vi "SaveForPrevious.vi"() -> ()   [LabVIEW 2016]
panel:
  out "error out":errorcluster
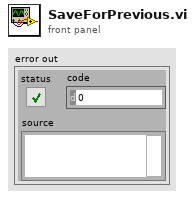
[diagram p1: front panel]
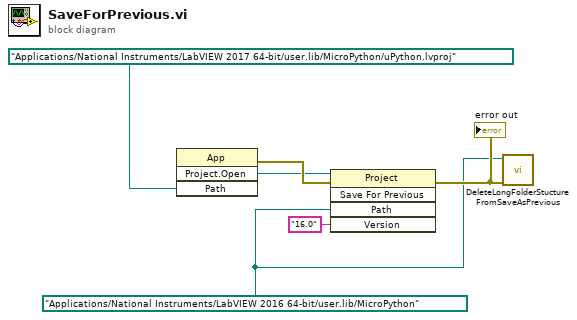
[diagram p0: block diagram]
diagram:
  w4 = path "/Applications/National Instruments/LabVIEW 2016 64-bit/user.lib/MicroPython" ("Path")
  n1 = invoke class="App" method="Project.Open"("Path"=path "/Applications/National Instruments/LabVIEW 2017 64-bit/user.lib/MicroPython/uPython.lvproj") -> (error out=w3:errorcluster, "Project:Open"=w2:refnum<vi>)  [unwired: 3 in, 2 out]
  n2 = invoke class="Project" method="Save For Previous"(reference=w2, error in=w3, "Path"=w4, "Version"="16.0") -> (error out=w5:errorcluster)  [unwired: 1 in, 4 out]
  "error out" <- w5
  n3 = call "DeleteLongFolderStuctureFromSaveAsPrevious.vi"("error in (no error)"=w5, "Path"=w4) -> ()  [unwired: 10 in]
